vi "Volts_to_temperature_(SubVI).vi"(4 "ch_data_string":string, 7 "error in":errorcluster, 16 "koeff. cluster":T1 {"k7" format="%#_18g"; "k6" format="%#_18g"; "k5" format="%#_18g"; "k4" format="%#_18g"; "k3" format="%#_18g"; "k2" format="%#_18g"; "k1" format="%#_18g"}) -> (9 "s? color":u32, 10 "Vin < 0?":bool, 20 "T solvation":dbl, 21 "meas_voltage":dbl, 27 "error out":errorcluster)   [LabVIEW 2015]
uses:
  <vilib>/express/express arith-compare/Formula/XNode/ExpressFormulaBlockNode.xnode
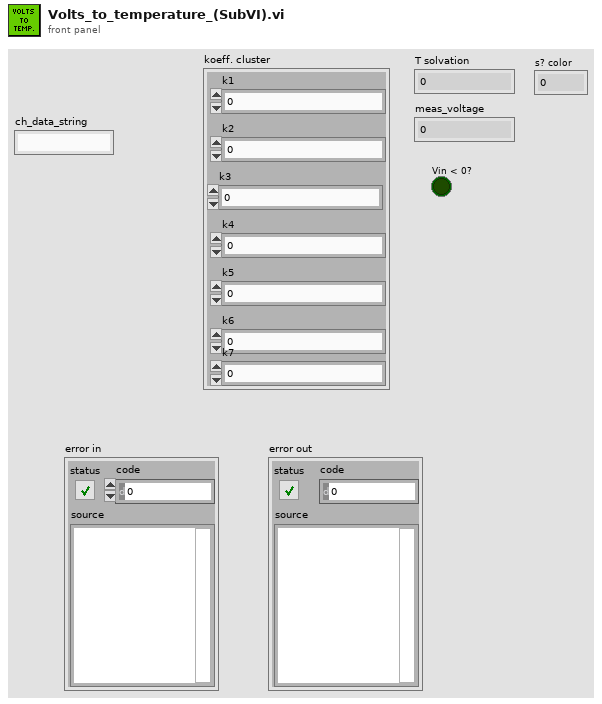
[diagram p1: front panel]
types:
  T1 = cluster{"k1":ext, "k2":ext, "k3":ext, "k4":ext, "k5":ext, "k6":ext, "k7":ext}
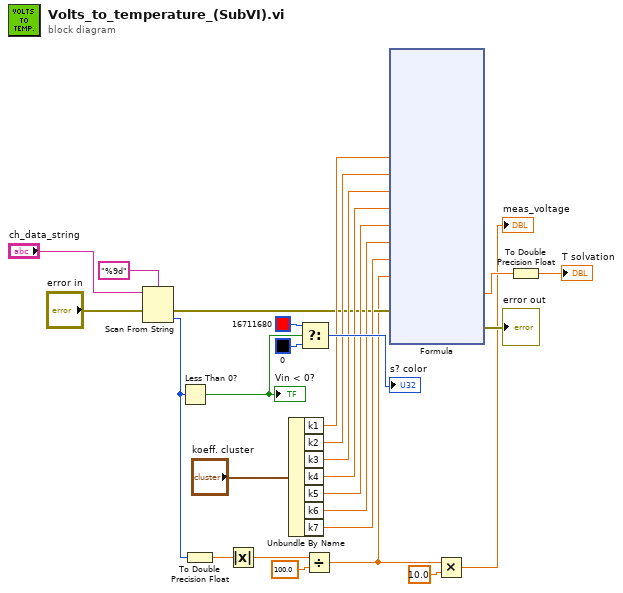
[diagram p0: block diagram]
diagram:
  n1 = Scan From String(format string="%9d", input string="ch_data_string", error in="error in") -> (error out=w11:errorcluster, output 1=w9:i32)  [unwired: 2 in, 2 out]
  n2 = Less Than 0?(x=w9) -> (x < 0?=w21:bool)
  "Vin < 0?" <- w21
  n3 = To Double Precision Float(number=w9) -> (double precision float=w19:dbl)
  n4 = Absolute Value(x=w19) -> (abs(x)=w7:dbl)
  n5 = Unbundle By Name("koeff. cluster") -> ("k1"=w18:ext, "k2"=w17:ext, "k3"=w16:ext, "k4"=w15:ext, "k5"=w14:ext, "k6"=w13:ext, "k7"=w12:ext)
  n6 = Select(t=u32 16711680, s=w21, f=u32 0) -> (s? t:f=→"s? color":u32)
  n7 = Divide(x=w7, y=100.0) -> (x/y=w2:dbl)
  n8 = xnode "Formula"("k1"=w18, "k2"=w17, "k3"=w16, "k4"=w15, "k5"=w14, "k6"=w13, "k7"=w12, "Rin"=w2, "error in (no error)"=w11) -> ("Result"=w5:ext, "error out"=→"error out":errorcluster)
  n9 = Multiply(x=w2, y=10.0) -> (x*y=→"meas_voltage":dbl)
  n10 = To Double Precision Float(number=w5) -> (double precision float=→"T solvation":dbl)
